vi "ABFLSHdll.vi"(8 "error in (no error)":errorcluster, 11 "Inputs":T1) -> (0 "error out":errorcluster, 3 "Outputs":T2)   [LabVIEW 2016]
doc: "subroutine ABFLSHdll(ab, a, b, z, iFlag, T, P, D, Dl, Dv, x, y, q, e, h, s, Cv, Cp, w, ierr, herr, ab_length,\nherr_length)\n\nGeneral flash calculation that handles all inputs of T, P, D, h, e, s, and q.\nThis includes both blind flash calculations, and situations where the phase is known to be liquid, vapor, or\n2-phase, and thus the calculation time will be much faster.\n\nMany of the 2-phase flash routines can accept initial estimates to decrease calculation time and increase convergence.\nABFLSH does not accept these, and ABFL2 or other routines will need to be called to use the initial estimates. These \nroutines end in the letters FL2.\n\nINPUTS:\nab -- Character string composed of two letters that indicate the input properties.\na -- Value of the property identified by the first letter in ab\nb -- Value of the property identified by the second letter in ab\nz -- Composition (array of mole fractions) For TQ and PQ inputs, send b=-99 for melting line states and b=-98 for sublimation line states.\niFlag -- Multiple flags combined into one variable (see above)\n\nOUTPUTS:\nT -- Temperature [K]\nP -- Pressure [kPa]\nD -- Density [mol/L or kg/m^3]\nDl -- Molar density of the liquid phase [mol/L or kg/m^3]\nDv -- Molar density of the vapor phase [mol/L or kg/m^3] If only one phase is present, Dl = Dv = D.\nx -- Composition of the liquid phase (array of mole or mass fractions)\ny -- Composition of the vapor phase (array of mole or mass fractions) If only one phase is present, x = y = z.\nq -- Vapor quality on a MOLAR basis (moles of vapor/total moles)\ne -- Overall internal energy [J/mol or kJ/kg]\nh -- Overall enthalpy [J/mol or kJ/kg]\ns -- Overall entropy [J/mol-K or kJ/kg-K]\nCv -- Isochoric (constant D) heat capacity [J/mol-K or kJ/kg-K]\nCp -- Isobaric (constant P) heat capacity [J/mol-K or kJ/kg-K]\nw -- Speed of sound [m/s]\nierr -- Error flag\nherr -- Error string (character*255)\nab_length -- length of variable ab (default: 2)\nherr_length -- length of variable herr (default: 255)"
uses:
  REFPROP.DLL
panel:
  # "REFPROP-ABSFLSHdll.vi"
  # "void  ABFLSHdll(CStr ab, double *a, double *b, double *z, double *T, double *P, double *D, double *Dl, double *Dv, double *x, double *y, double *q, double *e, double *h, double *s, double *Cv, double *Cp, double *w, int32_t *ierr, CStr herr, int32_t *ab_length, int32_t *herr_length);"
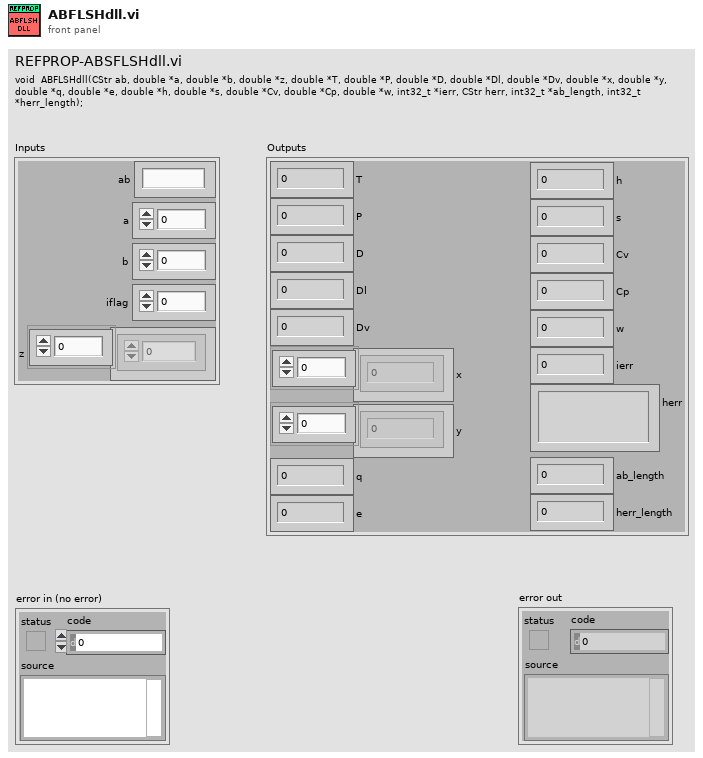
[diagram p1: front panel]
types:
  T1 = cluster{"ab":string, "a":dbl, "b":dbl, "iflag":i32, "z":dbl[]}
  T2 = cluster{"T":dbl, "P":dbl, "D":dbl, "Dl":dbl, "Dv":dbl, "x":dbl[], "y":dbl[], "q":dbl, "e":dbl, "h":dbl, "s":dbl, "Cv":dbl, "Cp":dbl, "w":dbl, "ierr":i32, "herr":string, "ab_length":i32, "herr_length":i32}
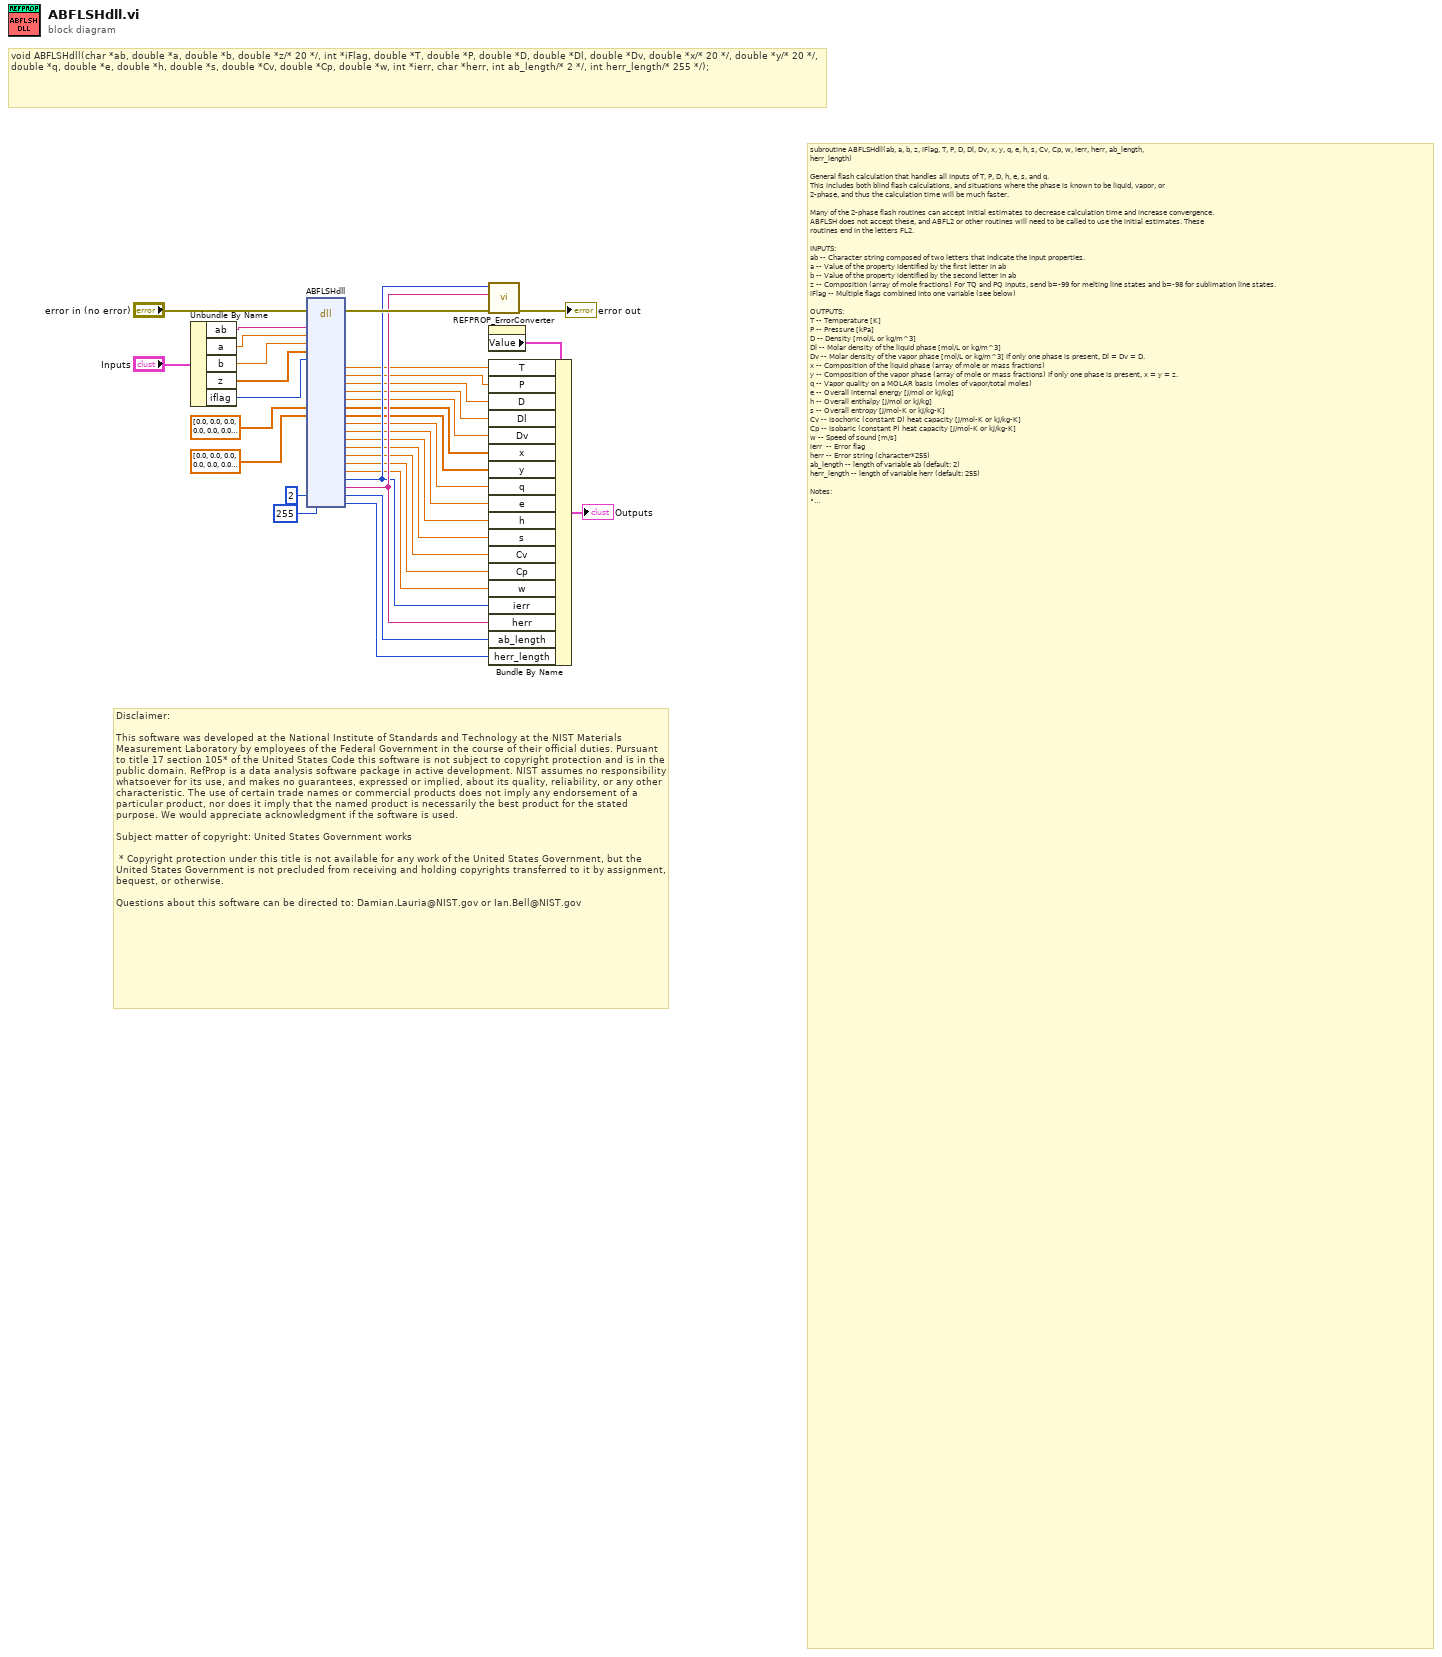
[diagram p0: block diagram]
diagram:
  # "void ABFLSHdll(char *ab, double *a, double *b, double *z/* 20 */, int *iFlag, double *T, double *P, double *D, double *Dl, double *Dv, double *x/* 20 */, double *y/* 20 */, double *q, double *e, double *h, double *s, double *Cv, double *Cp, double *w, int *ierr, char *herr, int ab_length/* 2 */, int herr_length/* 255 */);"
  # "Disclaimer:\n\nThis software was developed at the National Institute of Standards and Technology at the NIST Materials Measurement Laboratory by employees of the Federal Government in the course of their official duties. Pursuant to title 17 section 105* of the United States Code this software is not subject to copyright protection and is in the public domain. RefProp is a data analysis software package in active development. NIST assumes no responsibility whatsoever for its use, and makes no guarantees, expressed or implied, about its quality, reliability, or any other characteristic. The use of certain trade names or commercial products does not imply any endorsement of a particular product, nor does it imply that the named product is necessarily the best product for the stated purpose. We would appreciate acknowledgment if the software is used.\n \nSubject matter of copyright: United States Government works\n  \n * Copyright protection under this title is not available for any work of the United States Government, but the United States Government is not precluded from receiving and holding copyrights transferred to it by assignment, bequest, or otherwise.\n\nQuestions about this software can be directed to: Damian.Lauria@NIST.gov or Ian.Bell@NIST.gov"
  # "subroutine ABFLSHdll(ab, a, b, z, iFlag, T, P, D, Dl, Dv, x, y, q, e, h, s, Cv, Cp, w, ierr, herr, ab_length,\nherr_length)\n\nGeneral flash calculation that handles all inputs of T, P, D, h, e, s, and q.\nThis includes both blind flash calculations, and situations where the phase is known to be liquid, vapor, or\n2-phase, and thus the calculation time will be much faster.\n\nMany of the 2-phase flash routines can accept initial estimates to decrease calculation time and increase convergence.\nABFLSH does not accept these, and ABFL2 or other routines will need to be called to use the initial estimates. These \nroutines end in the letters FL2.\n\nINPUTS:\nab -- Character string composed of two letters that indicate the input properties.\na -- Value of the property identified by the first letter in ab\nb -- Value of the property identified by the second letter in ab\nz -- Composition (array of mole fractions) For TQ and PQ inputs, send b=-99 for melting line states and b=-98 for sublimation line states.\niFlag -- Multiple flags combined into one variable (see below)\n\nOUTPUTS:\nT -- Temperature [K]\nP -- Pressure [kPa]\nD -- Density [mol/L or kg/m^3]\nDl -- Molar density of the liquid phase [mol/L or kg/m^3]\nDv -- Molar density of the vapor phase [mol/L or kg/m^3] If only one phase is present, Dl = Dv = D.\nx -- Composition of the liquid phase (array of mole or mass fractions)\ny -- Composition of the vapor phase (array of mole or mass fractions) If only one phase is present, x = y = z.\nq -- Vapor quality on a MOLAR basis (moles of vapor/total moles)\ne -- Overall internal energy [J/mol or kJ/kg]\nh -- Overall enthalpy [J/mol or kJ/kg]\ns -- Overall entropy [J/mol-K or kJ/kg-K]\nCv -- Isochoric (constant D) heat capacity [J/mol-K or kJ/kg-K]\nCp -- Isobaric (constant P) heat capacity [J/mol-K or kJ/kg-K]\nw -- Speed of sound [m/s]\nierr  -- Error flag\nherr -- Error string (character*255)\nab_length -- length of variable ab (default: 2)\nherr_length -- length of variable herr (default: 255)\n\nNotes:\n• Cp and w are not defined for 2-phase states; the flag -9999980 is returned.\n• Cv for 2-phase states is not calculated (use CV2PK); the flag -9999990 is returned.\n\nInformation on ab\nValid character codes for ab are:\n• T - Temperature [K]\n• P - Pressure [kPa]\n• D - Density [mol/L or kg/m^3]\n• E - Internal energy [J/mol or kJ/kg]\n• H - Enthalpy [J/mol or kJ/kg]\n• S - Entropy [J/mol-K or kJ/kg]\n• Q - Quality [mol/mol or kJ/kg]\n• For example, ‘PH’ indicates pressure and enthalpy inputs.\n• For saturation properties, use codes of ‘TQ’ or ‘PQ’ for ab, and send b=1\n• The order of the letters does not matter, for example ‘DH’ = ‘HD’ for saturated vapor values and b=0 for\nsaturated liquid values.\n\nInformation on iFlags\nThree flags are currently allowed, and are sent combined in a three digit integer value. The digit on the right is\nthe mass flag (iMass) defined below, the middle digit is the phase flag (kph), and the digit on the left specifies\nother flags (k).\n• iMass: Molar or mass flag\n– 0 - All inputs and outputs are given on a mole basis.\n– 1 - All inputs and outputs are given on a mass basis.\n– 2 - All inputs and outputs are given on a mass basis except composition, which is given on a mole\nbasis.\n• kph: Phase flag (except for inputs of Q)\n– 0 - Unknown phase, the saturation routines will be called to determine the phase, which adds a\nsubstantial amount of time needed to calculate the properties.\n– 1 - State point is in the liquid phase, do not call saturation routine to determine state.\n– 2 - State point is in the vapor phase, do not call saturation routine to determine state.\n– 3 - State point is in the two-phase region.\n• kr,kq: Other flags for inputs of quality and either temperature or pressure (kq flag)\n– 1 - Quality on a molar basis (moles vapor/total moles) (default, the value of 1 is not necessarily\nneeded)\n– 2 - Quality on a mass basis (mass vapor/total mass); For inputs of T and either h or e (kr flag)\n6 Chapter 1. REFPROP DLL documentation\nREFPROP Documentation, Release 9.2\n– 3 - Return lower density root\n– 4 - Return higher density root\n\nExamples:\n• 000 - Default - Phase of state is unknown, molar units will be used everywhere, higher density root will be\nreturned.\n• 001 - Use mass based properties for everything except composition.\n• 011 - State is in the liquid, properties are mass based.\n• 300 - Return the lower density root for TH or TE inputs.\n• 200 - All inputs are on a mole basis, but quality is sent on a mass basis.\n\nFlags q flags\n\nq > 0 and q < 1 indicates a 2-phase state\nq < 0 Subcooled (compressed) liquid\nq = 0 Saturated liquid\nq = 1 Saturated vapor\nq > 1 Superheated vapor\nq = -998 Subcooled liquid, but quality not defined (usually P > Pc)\nq = 998 Superheated vapor, but quality not defined (usually T > Tc)\nq = 999 Supercritical state (T>Tc and P>Pc)"
  n1 = Unbundle By Name("Inputs") -> ("ab"=w9:string, "a"=w8:dbl, "b"=w7:dbl, "z"=w3:dbl[], "iflag"=w4:i32)
  n2 = dll-call lib="S:/009 - Testing/02 - Performance Testing/REFPROP/refprop.*" fn="ABFLSHdll"(error in="error in (no error)", "ab"=w9, "a"=w8, "b"=w7, "z"=w3, "iflag"=w4, "x"=dbl[] [0.0, 0.0, 0.0, 0.0, 0.0, 0.0, 0.0, 0.0, 0.0, 0.0, 0.0, 0.0, 0.0, 0.0, 0.0, 0.0, 0.0, 0.0, 0.0, 0.0] ("z"), "y"=dbl[] [0.0, 0.0, 0.0, 0.0, 0.0, 0.0, 0.0, 0.0, 0.0, 0.0, 0.0, 0.0, 0.0, 0.0, 0.0, 0.0, 0.0, 0.0, 0.0, 0.0] ("z"), "ab_length"=2, "herr_length"=255) -> (error out=w32:errorcluster, "T"=w12:dbl, "P"=w13:dbl, "D"=w14:dbl, "Dl"=w15:dbl, "Dv"=w16:dbl, "x"=w17:dbl[], "y"=w18:dbl[], "q"=w19:dbl, "e"=w20:dbl, "h"=w21:dbl, "s"=w22:dbl, "Cv"=w23:dbl, "Cp"=w24:dbl, "w"=w25:dbl, "ierr"=w26:i32, "herr"=w27:string, "ab_length"=w28:i32, "herr_length"=w29:i32)  [unwired: 22 in, 1 out]
  n3 = call "REFPROP_ErrorConverter.vi"("error in (no error)"=w32, "Error Message"=w27, "Error Code"=w26) -> ("error out"=→"error out":errorcluster)  [unwired: 8 in]
  n4 = property on="Outputs" class="Clust (strict)"() -> ("Value"=w30:T2)  [unwired: 2 in, 2 out]
  n5 = Bundle By Name(cluster=w30, "T"=w12, "P"=w13, "D"=w14, "Dl"=w15, "Dv"=w16, "x"=w17, "y"=w18, "q"=w19, "e"=w20, "h"=w21, "s"=w22, "Cv"=w23, "Cp"=w24, "w"=w25, "ierr"=w26, "herr"=w27, "ab_length"=w28, "herr_length"=w29) -> (→"Outputs":T2)
